vi "Exercise1.16-FIR Filter.vi"() -> ()   [LabVIEW 2013]
panel:
  out "Waveform Chart":cluster{"number: 0 to 1":dbl, dbl}(graph)
  in  "stop":bool
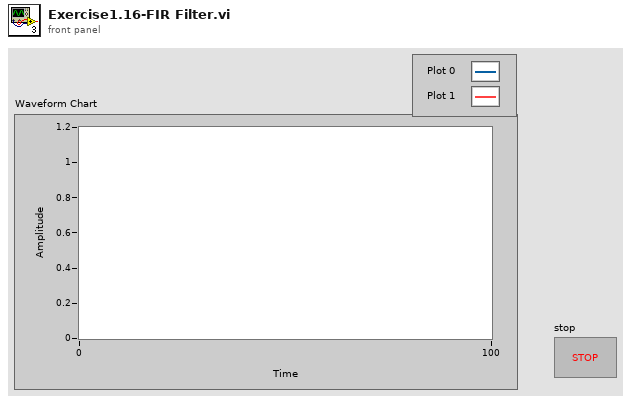
[diagram p1: front panel]
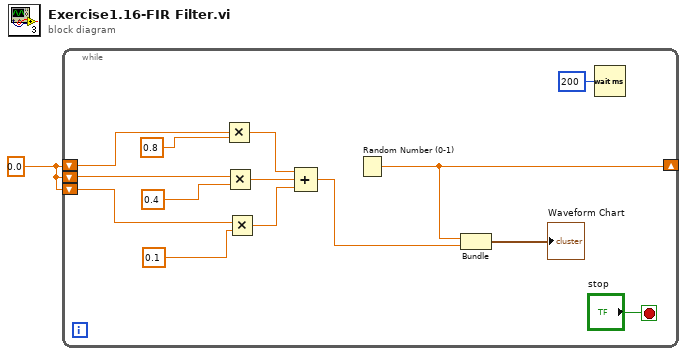
[diagram p0: block diagram]
diagram:
  w1 = 0.0
  n1 = while {
    shift-right: [w4] -> _
    shift-left: w1 -> [w15]
    shift-left: w1 -> [w10]
    shift-left: w1 -> [w11]
    stop <- "stop" stop-if-true
    n2 = Multiply(x=w15, y=0.8) -> (x*y=w7:dbl)
    n3 = Multiply(x=w11, y=0.4) -> (x*y=w8:dbl)
    n4 = Multiply(x=w10, y=0.1) -> (x*y=w9:dbl)
    n5 = Compound Arithmetic op=ADD(w7, w8, w9) -> (w3:dbl)
    n6 = Random Number (0-1)() -> (number: 0 to 1=w4:dbl)
    n7 = Bundle("number: 0 to 1"=w4, w3) -> (→"Waveform Chart":cluster{"number: 0 to 1":dbl, dbl})  [unwired: 1 in]
    n8 = Wait (ms)(milliseconds to wait=u32 200) -> ()  [unwired: 1 out]
  }
